vi "Set Acquired Samples Counter.vi"(9 "Set":bool, 10 "Set":u16) -> (2 "Value":u16)   [LabVIEW 2011]
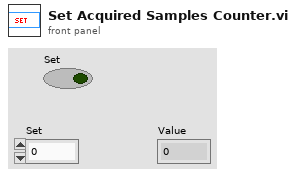
[diagram p1: front panel]
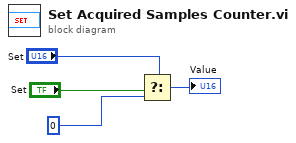
[diagram p0: block diagram]
diagram:
  n1 = Select(t="Set", s="Set", f=u16 0) -> (s? t:f=→"Value":u16)
